vi "extract_carriers.vi"(4 "Noise floor":dbl[][](array[numeric]) format="%#_6p", 5 "Trace info":T1, 6 "Spectrum":waveform(cdb)[](array[waveform]), 7 "Level selector":T4, 8 "Ref carrier amplitudes":cdb[][][](array[numeric]) format="%#_3p", 9 "Modulation info":T15={"Fs full"=0.0, "Fs high"=0.0, "Fs low"=0.0, "Read size"=0, "FFT size low"=5000, "df low"=5000.0, "High carriers"=[], "Low carriers"=[], "Hi channels at low"=[7]} {"Hi channels at low" min=0 step=1; "Low carriers" format="%#_6p"; "High carriers" format="%#_6p"}, 10 "Config":T9={"IO params"={"Conversion"={"Rate"=4.0, "In channels"=2, "Out channels"=4}, "Carriers"={"Phase shift"=180.0, "Levels"=[[0.8, 0.8, 0.8], [0.03, 0.03, 0.03]], "Delay samples"=73.15}}, "High rate STFT"={"Win param"=101.5, "Window type"=61, "Win order"=2, "DFT size"=64, "Channels"=[7], "Oversample"=64}, "Low rate STFT"={"Win param"=120.0, "Window type"=61, "Win order"=8, "DFT size"=64, "Channels"=[7], "Oversample"=64}, "Filtering"={"Hum"={"Frequency"=0.0, "Tc"=0.0, "Limit"=101.5, "FFT filter"=FALSE, "Detrend mode"=enum."Robust linear", "Enable"=FALSE}, "Kalman"={"Process noise"=101.5, "Measure noise"=101.5, "Unlock m noise"=101.5, "Mode"=enum."FFT"}, "Distortion"={"LF cut"=101.5, "Tc"=3.0, "Limit"=101.5, "FFT filter"=FALSE, "Detrend mode"=enum."Robust linear", "Enable"=FALSE}, "Lowpass"={"Frequency"=0.0, "Order"=0, "Enable"=FALSE}, "Impulse"={"Win order"=102, "Locked limit"=101.5, "Locked count"=102, "Threshold Tc"=101.5, "Thresh sigmas"=101.5, "Thresh min"=101.5, "After"=0, "Detrend"=FALSE, "Enable"=FALSE}}} {"Filtering"."Impulse"."Thresh min" format="%#_3p"; "Filtering"."Impulse"."Threshold Tc" format="%#_3p"; "Filtering"."Impulse"."Locked limit" format="%#_3p"; "Filtering"."Impulse"."Thresh sigmas" format="%#_3p"; "Filtering"."Lowpass"."Frequency" format="%#_4p"; "Filtering"."Distortion"."Limit" format="%#_3p"; "Filtering"."Distortion"."LF cut" format="%#_3p"; "Filtering"."Kalman"."Unlock m noise" format="%#_3p"; "Filtering"."Kalman"."Measure noise" format="%#_3p"; "Filtering"."Kalman"."Process noise" format="%#_3p"; "Filtering"."Hum"."Limit" format="%#_3p"; "Filtering"."Hum"."Frequency" format="%#_4p"; "Low rate STFT"."Oversample" min=1 step=1; "Low rate STFT"."Channels" min=0 step=1; "Low rate STFT"."DFT size" min=1 step=1; "Low rate STFT"."Window type" items=["Rectangle"=0, "Hanning"=1, "Hamming"=2, "Blackman-Harris"=3, "Exact Blackman"=4, "Blackman"=5, "Flat Top"=6, "4 Term B-Harris "=7, "7 Term B-Harris"=8, "Low Sidelobe"=9, "Blackman Nuttall"=11, "Triangle"=30, "Bartlett-Hanning"=31, "Bohman"=32, "Parzen"=33, "Welch"=34, "Kaiser"=60, "Dolph-Chebyshev"=61, "Gaussian"=62]; "High rate STFT"."Oversample" min=1 step=1; "High rate STFT"."Channels" min=0 step=1; "High rate STFT"."DFT size" min=1 step=1; "High rate STFT"."Window type" items=["Rectangle"=0, "Hanning"=1, "Hamming"=2, "Blackman-Harris"=3, "Exact Blackman"=4, "Blackman"=5, "Flat Top"=6, "4 Term B-Harris "=7, "7 Term B-Harris"=8, "Low Sidelobe"=9, "Blackman Nuttall"=11, "Triangle"=30, "Bartlett-Hanning"=31, "Bohman"=32, "Parzen"=33, "Welch"=34, "Kaiser"=60, "Dolph-Chebyshev"=61, "Gaussian"=62]; "IO params"."Carriers"."Levels" min=0.0 step=0.1; "IO params"."Conversion"."Rate" format="%#_8g"}, 11 "Carrier amplitudes":cdb[][][](array[numeric]) format="%#_3p") -> (3 "Levels":dbl[][](array[numeric]) format="%.3f")   [LabVIEW 2014]
uses:
  modulation_info.ctl
  ilemt_config.ctl
  IO_params.ctl
  stft_params.ctl
  <vilib>/Analysis/4window.llb/windowTd.ctl
  filter_params.ctl
  detrend_mode.ctl
  levels_selector.ctl
  Level selector 1.ctl
  Level selector 4.ctl
  Level selector 3.ctl
  Level selector 2.ctl
  trace_info.ctl
  trace_channel.ctl
  ilemt_status.ctl
  <vilib>/Analysis/NI_AALPro.lvlib
panel:
  # "High"
  # "Low"
  # "X"
  # "Y"
  # "Z"
  # "First dimension (page) is measure/sense selector"
  # "High"
  # "Low"
  # "X"
  # "Y"
  # "Z"
  # "High"
  # "Low"
  # "X"
  # "Y"
  # "Z"
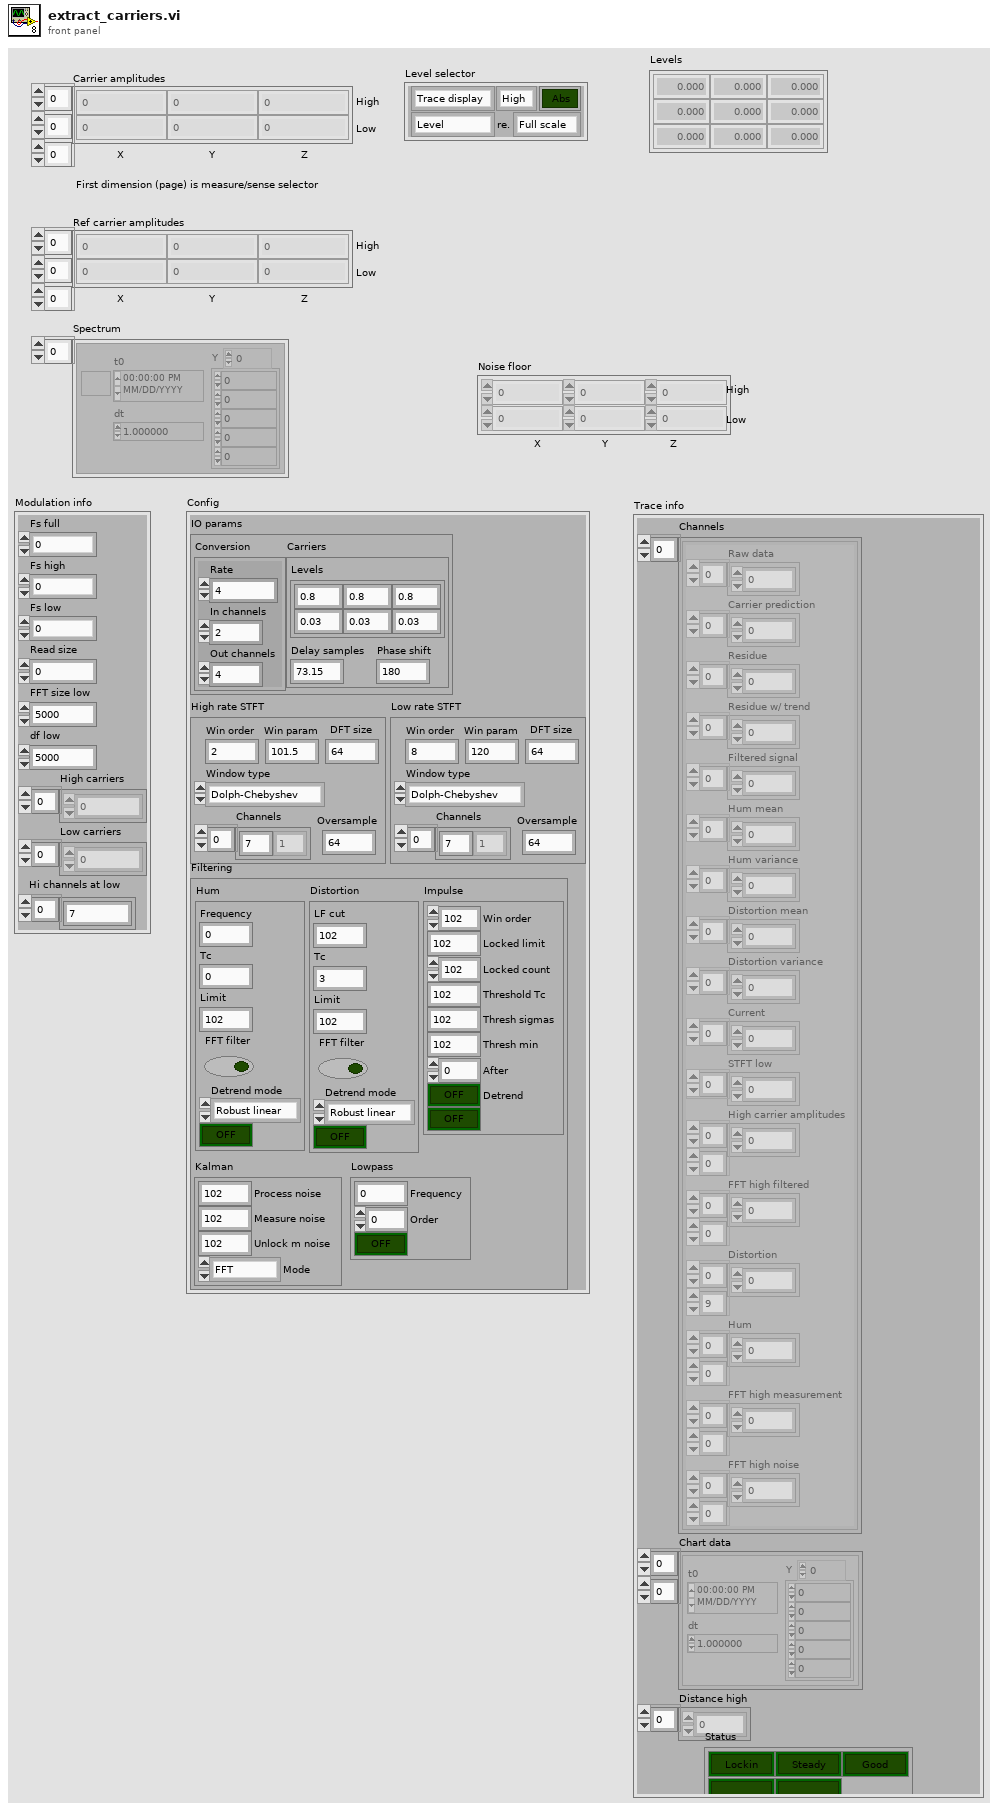
[diagram p1: front panel]
types:
  T1 = typedef "trace_info.ctl" = cluster{"Channels":T2[], "Chart data":waveform(dbl)[][], "Distance high":dbl[], "Status":T3}
  T2 = typedef "trace_channel.ctl" = cluster{"Raw data":dbl[], "Carrier prediction":dbl[], "Residue":dbl[], "Residue w/ trend":dbl[], "Filtered signal":dbl[], "Hum mean":dbl[], "Hum variance":dbl[], "Distortion mean":dbl[], "Distortion variance":dbl[], "Current":dbl[], "STFT low":cdb[], "High carrier amplitudes":cdb[][], "FFT high filtered":cdb[][], "Distortion":cdb[][], "Hum":cdb[][], "FFT high measurement":cdb[][], "FFT high noise":dbl[][]}
  T3 = typedef "ilemt_status.ctl" = cluster{"Unlocked":bool, "Impulse":bool, "NaN":bool, "Backlog":bool, "Clipping":bool}
  T4 = typedef "levels_selector.ctl" = cluster{"Signal source":T5, "Mode":T6, "re.":T7, "High/low":T8, "Sense":bool}
  T5 = typedef "Level selector 1.ctl" = enum16{"Trace display", "Carrier levels", "Ref levels", "Distortion"}
  T6 = typedef "Level selector 4.ctl" = enum16{"Level", "dB", "Phase", "Mismatch"}
  T7 = typedef "Level selector 3.ctl" = enum16{"Full scale", "Carrier", "Ref level", "Noise"}
  T8 = typedef "Level selector 2.ctl" = enum16{"High", "Low"}
  T9 = typedef "ilemt_config.ctl" = cluster{"IO params":T10, "High rate STFT":T11, "Low rate STFT":T11, "Filtering":T13}
  T10 = typedef "IO_params.ctl" = cluster{"Conversion":cluster{"Rate":dbl, "In channels":u32, "Out channels":u32}, "Carriers":cluster{"Phase shift":dbl, "Levels":dbl[][], "Delay samples":dbl}}
  T11 = typedef "stft_params.ctl" = cluster{"Win param":dbl, "Window type":T12, "Win order":i32, "DFT size":i32, "Channels":i32[], "Oversample":i32}
  T12 = typedef "NI_AALPro.lvlib/windowTd.ctl" = u32
  T13 = typedef "filter_params.ctl" = cluster{"Hum":cluster{"Frequency":dbl, "Tc":dbl, "Limit":dbl, "FFT filter":bool, "Detrend mode":T14, "Enable":bool}, "Kalman":cluster{"Process noise":dbl, "Measure noise":dbl, "Unlock m noise":dbl, "Mode":enum16{"FFT", "KF demod"}}, "Distortion":cluster{"LF cut":dbl, "Tc":dbl, "Limit":dbl, "FFT filter":bool, "Detrend mode":T14, "Enable":bool}, "Lowpass":cluster{"Frequency":dbl, "Order":i32, "Enable":bool}, "Impulse":cluster{"Win order":i32, "Locked limit":dbl, "Locked count":i32, "Threshold Tc":dbl, "Thresh sigmas":dbl, "Thresh min":dbl, "After":i32, "Detrend":bool, "Enable":bool}}
  T14 = typedef "detrend_mode.ctl" = enum16{"Zero mean", "Linear", "Robust linear"}
  T15 = typedef "modulation_info.ctl" = cluster{"Fs full":dbl, "Fs high":dbl, "Fs low":dbl, "Read size":i32, "FFT size low":i32, "df low":dbl, "High carriers":dbl[], "Low carriers":dbl[], "Hi channels at low":i32[]}
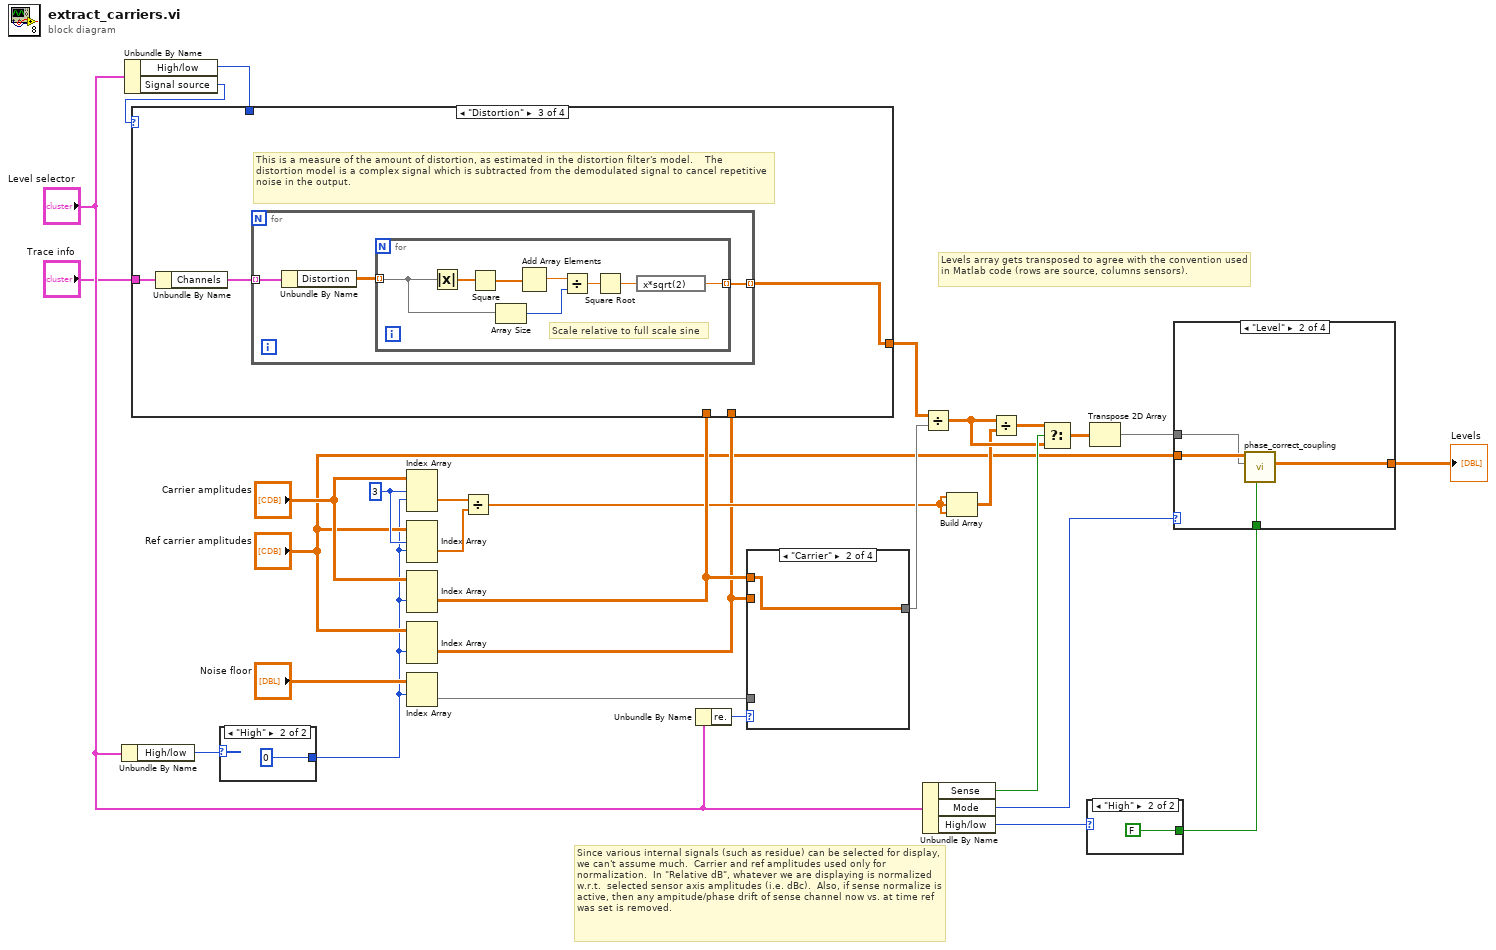
[diagram p0: block diagram]
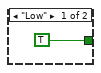
[diagram p2: hidden frame]
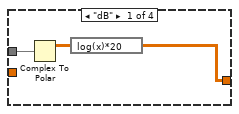
[diagram p3: hidden frame]
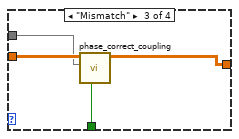
[diagram p4: hidden frame]
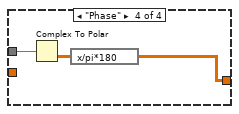
[diagram p5: hidden frame]
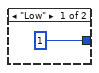
[diagram p6: hidden frame]
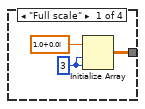
[diagram p7: hidden frame]
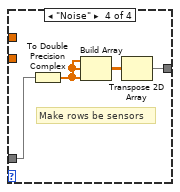
[diagram p9: hidden frame]
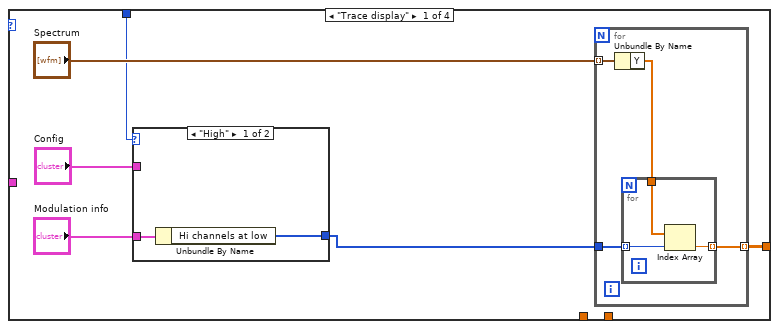
[diagram p10: hidden frame]
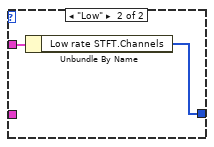
[diagram p11: hidden frame]
diagram:
  w20 = 3 ("disabled index (page)")
  # "Levels array gets transposed to agree with the convention used in Matlab code (rows are source, columns sensors)."
  # "Since various internal signals (such as residue) can be selected for display, we can't assume much.  Carrier and ref amplitudes used only for normalization.  In \"Relative dB\", whatever we are displaying is normalized w.r.t.  selected sensor axis amplitudes (i.e. dBc).  Also, if sense normalize is active, then any ampitude/phase drift of sense channel now vs. at time ref was set is removed."
  n1 = Unbundle By Name("Level selector") -> ("High/low"=w26:T8)
  n2 = Unbundle By Name("Level selector") -> ("High/low"=w28:T8, "Signal source"=w29:T5)
  n3 = case shown="\"High\"" w26 {
    tunnel: [1 0] -> w3
    frame "Low" {
    }
    frame "High" {
    }
  }
  n4 = Index Array(array="Carrier amplitudes", index (dim 0)=w20, index (dim 1)=w3) -> (element=w19:cdb[])  [unwired: 1 in]
  n5 = Index Array(array="Ref carrier amplitudes", index (dim 0)=w20, index (dim 1)=w3) -> (element=w18:cdb[])  [unwired: 1 in]
  n6 = Index Array(array="Carrier amplitudes", index (dim 1)=w3) -> (element=w22:cdb[][])  [unwired: 2 in]
  n7 = Index Array(array="Ref carrier amplitudes", index (dim 1)=w3) -> (element=w11:cdb[][])  [unwired: 2 in]
  n8 = case shown="\"Distortion\"" w29 {
    tunnel: [w34 w49 w50 w64] -> w25
    tunnel: w28 -> [w35 _ _ _]
    tunnel: w22 -> [_ w49 _ _]
    tunnel: w11 -> [_ _ _ w64]
    tunnel: "Trace info" -> [_ _ w52 _]
    frame "Trace display" {
      n9 = case shown="\"High\"" w35 {
        tunnel: [w45 w47] -> w32
        tunnel: "Config" -> [_ w48]
        tunnel: "Modulation info" -> [w46 _]
        frame "High" {
          n10 = Unbundle By Name(w46) -> ("Hi channels at low"=w45:i32[])
        }
        frame "Low" {
          n11 = Unbundle By Name(w48) -> ("Low rate STFT.Channels"=w47:i32[])
        }
      }
      n12 = for {
        tunnel: "Spectrum" -> [w39] mode=indexing
        tunnel: w32 -> [w41]
        tunnel: [w40] -> w34 mode=indexing
        n13 = Unbundle By Name(w39) -> ("Y"=w38:cdb[])
        n14 = for {
          tunnel: w41 -> [w42] mode=indexing
          tunnel: w38 -> [w44]
          tunnel: [w43] -> w40 mode=indexing
          n15 = Index Array(array=w44, index=w42) -> (element=w43:cdb)
        }
      }
    }
    frame "Carrier levels" {
    }
    frame "Distortion" {
      # "This is a measure of the amount of distortion, as estimated in the distortion filter's model.    The distortion model is a complex signal which is subtracted from the demodulated signal to cancel repetitive noise in the output."
      n16 = Unbundle By Name(w52) -> ("Channels"=w51:T2[])
      n17 = for {
        tunnel: w51 -> [w55] mode=indexing
        tunnel: [w54] -> w50 mode=indexing
        n18 = Unbundle By Name(w55) -> ("Distortion"=w53:cdb[][])
        n19 = for {
          tunnel: w53 -> [w59] mode=indexing
          tunnel: [w56] -> w54 mode=indexing
          # "Scale relative to full scale sine"
          n20 = Absolute Value(x=w59) -> (abs(x)=w58:dbl[])
          n21 = Square(x=w58) -> (x^2=w63:dbl[])
          n22 = Array Size(array=w59) -> (size(s)=w60:i32)
          n23 = Add Array Elements(numeric array=w63) -> (sum=w62:dbl)
          n24 = Divide(x=w62, y=w60) -> (x/y=w61:dbl)
          n25 = Square Root(x=w61) -> (sqrt(x)=w57:dbl)
          n26 = expression code="x*sqrt(2)"(w57) -> (w56:dbl)
        }
      }
    }
    frame "Ref levels" {
    }
  }
  n27 = Index Array(array="Noise floor", index (row)=w3) -> (element=w2:dbl[])  [unwired: 1 in]
  n28 = Divide(x=w19, y=w18) -> (x/y=w13:cdb[])
  n29 = Unbundle By Name("Level selector") -> ("re."=w27:T7)
  n30 = case shown="\"Carrier\"" w27 {
    tunnel: w22 -> [_ w68 _ _]
    tunnel: [w65 w68 w69 w70] -> w24
    tunnel: w11 -> [_ _ w69 _]
    tunnel: w2 -> [_ _ _ w73]
    frame "Full scale" {
      w66 = 3 ("dimension size")
      n31 = Initialize Array(cdb 1.0+0.0i, w66, w66) -> (w65:cdb[][])
    }
    frame "Carrier" {
    }
    frame "Ref level" {
    }
    frame "Noise" {
      # "Make rows be sensors"
      n32 = To Double Precision Complex(1:w73) -> (0:w72:cdb[])
      n33 = Build Array(w72, w72, w72) -> (w71:cdb[][])
      n34 = Transpose 2D Array(2D array=w71) -> (transposed array=w70:cdb[][])
    }
  }
  n35 = Divide(x=w25, y=w24) -> (x/y=w15:cdb[][])
  n36 = Unbundle By Name("Level selector") -> ("Sense"=w17:bool, "Mode"=w14:T6, "High/low"=w8:T8)
  n37 = Build Array(w13, w13, w13) -> (w12:cdb[][])
  n38 = Divide(x=w15, y=w12) -> (x/y=w16:cdb[][])
  n39 = Select(t=w16, s=w17, f=w15) -> (s? t:f=w6:cdb[][])
  n40 = case shown="\"High\"" w8 {
    tunnel: [TRUE FALSE] -> w7
    frame "Low" {
    }
    frame "High" {
    }
  }
  n41 = Transpose 2D Array(2D array=w6) -> (transposed array=w5:cdb[][])
  n42 = case shown="\"Level\"" w14 {
    tunnel: w5 -> [w78 w79 w84 w88]
    tunnel: [w76 w81 w83 w87] -> w9
    tunnel: "Ref carrier amplitudes" -> [_ w82 w86 _]
    tunnel: w7 -> [_ w80 w85 _]
    frame "dB" {
      n43 = Complex To Polar(r * e^(i*theta)=w78) -> (r=w77:dbl[][])  [unwired: 1 out]
      n44 = expression code="log(x)*20"(w77) -> (w76:dbl[][])
    }
    frame "Level" {
      n45 = call "phase_correct_coupling.vi"("Is low?"=w80, "Complex coupling"=w79, "Ref carrier ampl"=w82) -> ("Phase corrected coupling"=w81:cdb[][])  [unwired: 7 in, 1 out]
    }
    frame "Mismatch" {
      n46 = call "phase_correct_coupling.vi"("Is low?"=w85, "Complex coupling"=w84, "Ref carrier ampl"=w86) -> ("Phase mismatch"=w83:dbl[][])  [unwired: 7 in, 1 out]
    }
    frame "Phase" {
      n47 = Complex To Polar(r * e^(i*theta)=w88) -> (theta=w89:dbl[][])  [unwired: 1 out]
      n48 = expression code="x/pi*180"(w89) -> (w87:dbl[][])
    }
  }
  "Levels" <- w9
